vi "getLaserCmmd.vi"(1 "Cmmd index":i32=1, 2 "Laser type":i32) -> (0 "Laser command":string="?LOf")   [LabVIEW 2015]
panel:
  in  "Laser commands":string[][](array[string])=[["?LOn", "?LOf", "?SLP"], ["SOURce:AM:STATe ON ", "SOURce:AM:STATe OFF ", "SOURce:POWer:LEVel:IMMediate:AMPLitude "]]
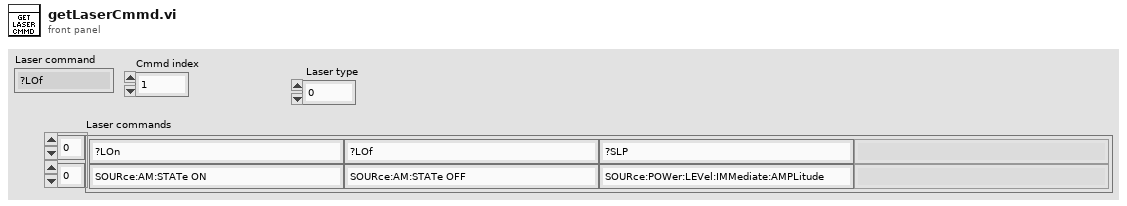
[diagram p1: front panel]
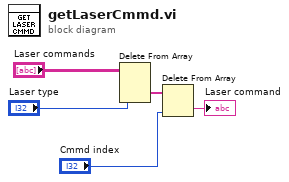
[diagram p0: block diagram]
diagram:
  n1 = Delete From Array(array="Laser commands", index (row)="Laser type") -> (deleted portion=w3:string[])  [unwired: 2 in, 1 out]
  n2 = Delete From Array(array=w3, index="Cmmd index") -> (deleted portion=→"Laser command":string)  [unwired: 1 in, 1 out]
